vi "Change Version_VI Version.vi"() -> ()   [LabVIEW 2020, in "PPL Version Issue.lvlib"]
uses:
  PPL Version Issue.lvlib
  <vilib>/AppBuilder/AB_API_Simple/Build Specification Version.ctl
  <vilib>/AppBuilder/AB_API_Simple/Get Build Specification Version (path).vi
  <vilib>/AppBuilder/AB_API_Simple/Set Build Specification Version (path).vi
  <vilib>/AppBuilder/AB_API_Simple/NI_App_Builder_API.lvlib
panel:
  in  "Build Specification Version to set":T1
  out "error out":errorcluster
  out "Build Specification Version":T1
  # "Read first then write... so call twice to verify your change..."
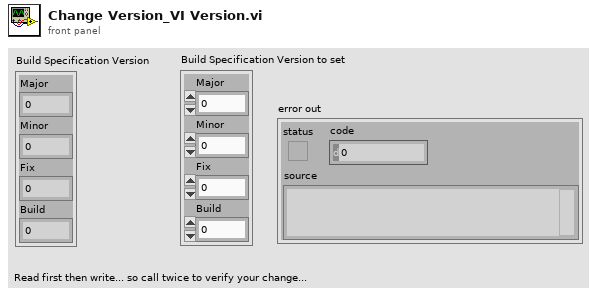
[diagram p1: front panel]
types:
  T1 = typedef "NI_App_Builder_API.lvlib/Build Specification Version.ctl" = cluster{"Major":u16, "Minor":u16, "Fix":u16, "Build":u16}
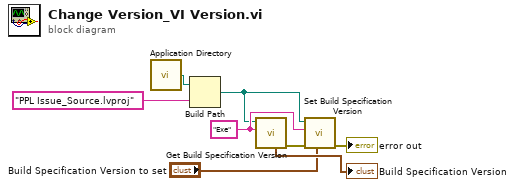
[diagram p0: block diagram]
diagram:
  w4 = "Exe" ("Name of build specification")
  n1 = call <vilib>:"Application Directory.vi"() -> ("Application Directory"=w1:path)
  n2 = Build Path(base path=w1, name or relative path="PPL Issue_Source.lvproj") -> (appended path=w2:path)
  n3 = call-poly <vilib>:"Get Build Specification Version.vi"("Name of build specification"=w4, "Path to project"=w2) -> ("error out"=w5:errorcluster, "Build Specification Version"=→"Build Specification Version":T1)  [unwired: 8 in]
  n4 = call-poly <vilib>:"Set Build Specification Version.vi"("Build Specification Version"="Build Specification Version to set", "error in (no error)"=w5, "Name of build specification"=w4, "Path to project"=w2) -> ("error out"=→"error out":errorcluster)  [unwired: 7 in]
